vi "Create (String).vi"(8 "error in (no error)":errorcluster) -> (0 "error out":errorcluster, 3 "URI out":refnum<class "URI.lvclass">)   [LabVIEW 2020, in "URI.lvlib" / "URI.lvclass"]
uses:
  URI.lvclass
  URI.lvclass/URI.ctl
  URI.lvlib
panel:
  in  "URI String":string
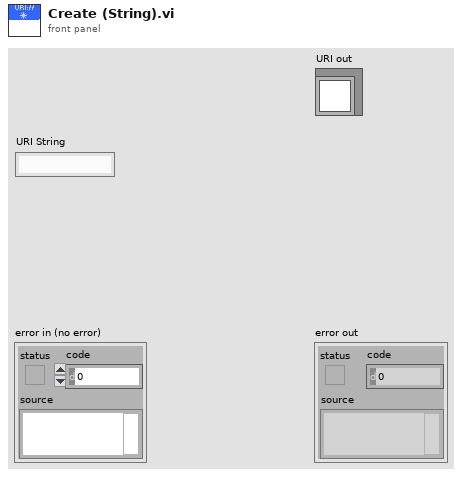
[diagram p1: front panel]
types:
  T1 = typedef "URI.lvlib/URI Components.ctl" = cluster{"Scheme":string, "User Info":string, "Host":string, "Port":string, "Path":string, "Query":string, "Fragment":string}
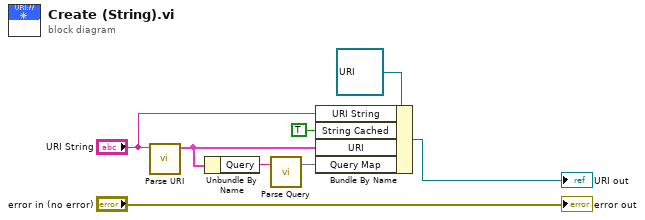
[diagram p0: block diagram]
diagram:
  n1 = call "Parse URI.vi"("URI String"="URI String") -> ("Parsed Components"=w3:T1)  [unwired: 9 in, 1 out]
  n2 = Unbundle By Name(w3) -> ("Query"=w2:string)
  n3 = call "Parse Query.vi"("Query String"=w2) -> ("Query Map"=w1:map{string, string})  [unwired: 6 in]
  n4 = Bundle By Name(cluster=refnum<class "URI.lvclass"> refnum ("URI in"), "URI String"="URI String", "String Cached"=TRUE, "URI"=w3, "Query Map"=w1) -> (→"URI out":refnum<class "URI.lvclass">)
  "error out" <- "error in (no error)"
